vi "SSL Detection Frame Balls Estimator.vi"(5 "Time Stamp":timestamp, 7 "Life Time":dbl=1.0, 10 "dt":dbl, 11 "Balls":T1[](array[typedef])) -> (3 "Est balls":T1[](array[typedef]))   [LabVIEW 2018]
uses:
  SSL Detection Ball.ctl
  <vilib>/Analysis/Matrix/Datatypes/RealMatrix.ctl
  <vilib>/Analysis/Matrix/NI_Matrix.lvlib
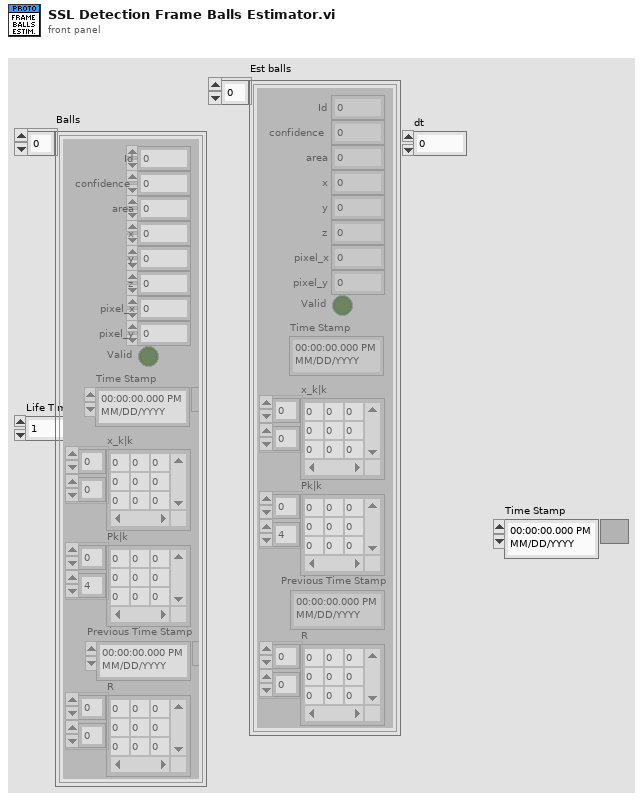
[diagram p1: front panel]
types:
  T1 = typedef "SSL Detection Ball.ctl" = cluster{"x":sgl, "area":u32, "confidence":sgl, "y":sgl, "z":sgl, "pixel_x":sgl, "pixel_y":sgl, "Valid":bool, "Time Stamp":timestamp, "x_k|k":T2, "Pk|k":T2, "Id":u32, "Previous Time Stamp":timestamp, "R":T2}
  T2 = typedef "NI_Matrix.lvlib/RealMatrix.ctl" = dbl[][]
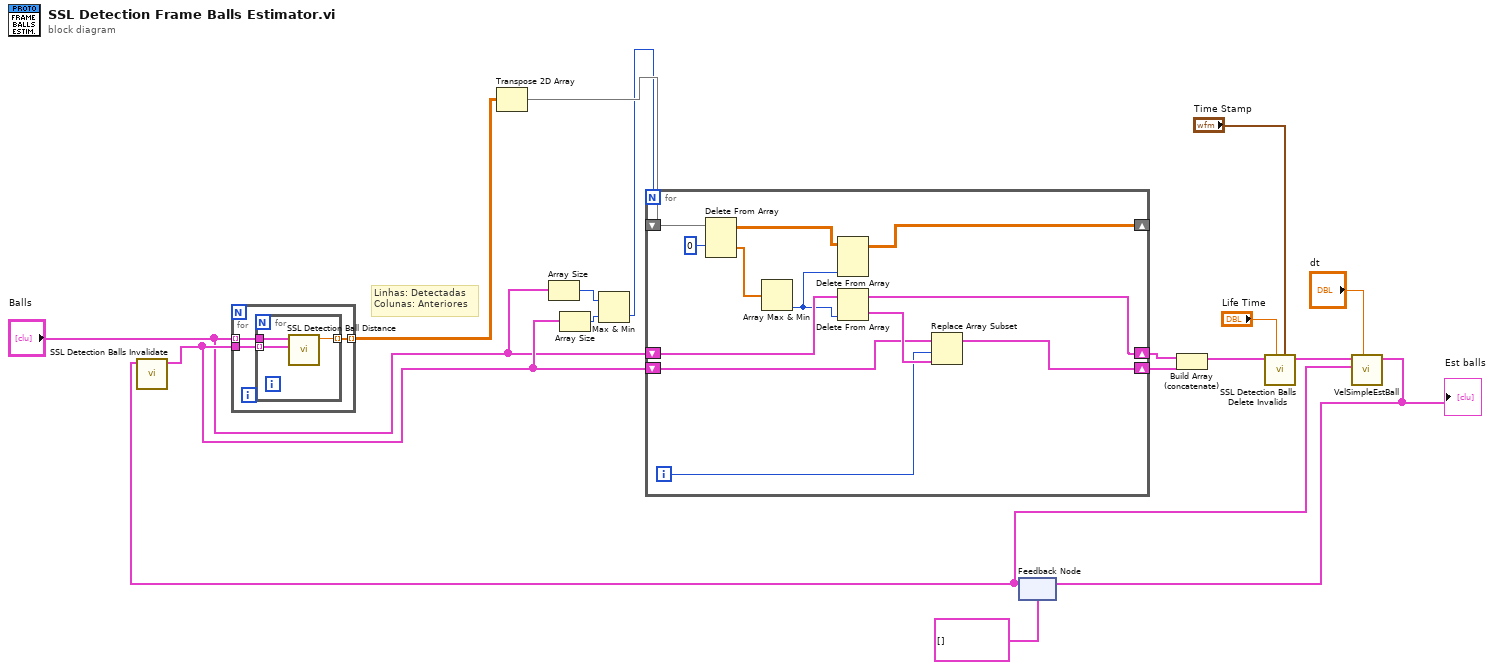
[diagram p0: block diagram]
diagram:
  # "Linhas: Detectadas\nColunas: Anteriores"
  n1 = Array Size(array="Balls") -> (size(s)=w11:i32)
  n2 = feedback #1(T1[] [] ("Balls Out")) -> (w3:T1[])
  n3 = call "SSL Detection Balls Invalidate.vi"("Value"=w3) -> ("Array"=w15:T1[])  [unwired: 10 in]
  n4 = for {
    tunnel: "Balls" -> [w20] mode=indexing
    tunnel: w15 -> [w19]
    tunnel: [w18] -> w17 mode=indexing
    n5 = for {
      tunnel: w20 -> [w23]
      tunnel: w19 -> [w22] mode=indexing
      tunnel: [w21] -> w18 mode=indexing
      n6 = call "SSL Detection Ball Distance.vi"("Detection Ball"=w22, "Detection Ball 2"=w23) -> ("norm"=w21:dbl)  [unwired: 9 in]
    }
  }
  n7 = Transpose 2D Array(2D array=w17) -> (transposed array=w16:dbl[][])
  n8 = Array Size(array=w15) -> (size(s)=w10:i32)
  n9 = Max & Min(x=w11, y=w10) -> (min(x,y)=w9:i32)  [unwired: 1 out]
  n10 = for {
    N: w9 -> [_]
    shift-right: [w29] -> w13
    shift-left: w15 -> [w30]
    shift-right: [w26] -> _
    shift-left: w16 -> [w35]
    shift-right: [w24] -> w14
    shift-left: "Balls" -> [w32]
    i -> [w28]
    n11 = Delete From Array(array=w35, index (row)=0) -> (deleted portion=w33:dbl[], array with subset deleted=w27:dbl[][])  [unwired: 2 in]
    n12 = Array Max & Min(array=w33) -> (min index (indices)=w25:i32)  [unwired: 3 out]
    n13 = Delete From Array(array=w27, index (col)=w25) -> (array with subset deleted=w26:dbl[][])  [unwired: 2 in, 1 out]
    n14 = Delete From Array(array=w32, index=w25) -> (deleted portion=w31:T1, array with subset deleted=w24:T1[])  [unwired: 1 in]
    n15 = Replace Array Subset(array=w30, new element=w31, index=w28) -> (w29:T1[])
  }
  n16 = Build Array (concatenate)(w14, w13) -> (w12:T1[])
  n17 = call "SSL Detection Balls Delete Invalids.vi"("Now"="Time Stamp", "Life Time"="Life Time", "Balls In"=w12) -> ("Balls Out"=w4:T1[])  [unwired: 8 in]
  n18 = call "VelSimpleEstBall.vi"("dt"="dt", "Balls Out"=w3, "Balls Out 2"=w4) -> ("Array"=w2:T1[])  [unwired: 8 in]
  "Est balls" <- w2
  n19 = feedback-in #1(w2) -> ()
